vi "Laurel Meter Serial.vi"(8 "error in (no error)":errorcluster, 10 "VISA resource name":refnum<visa-resource-name>, 11 "Send Command":T1(ring)) -> (0 "error out":errorcluster, 3 "Output":dbl format="%.2f")   [LabVIEW 2012]
panel:
  out "return count":u32
  out "read buffer":string
  out "Numeric":i32
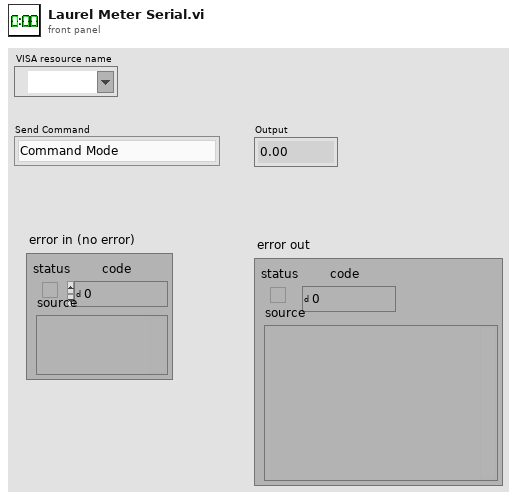
[diagram p1: front panel]
types:
  T1 = enum16{"Command Mode", "Cold Reset", "Function Reset", "Reading: All Active Items", "Reading: Item 1", "Reading: Item 2", "Reading: Item 3"}
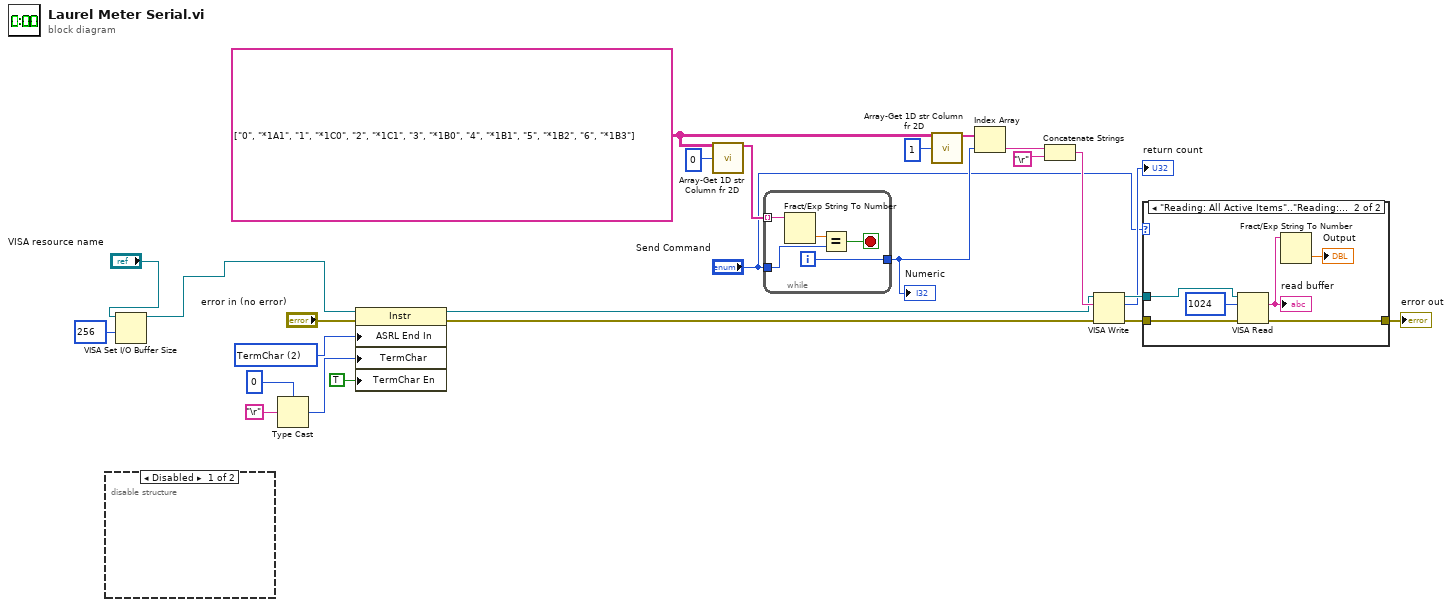
[diagram p0: block diagram]
diagram:
  w14 = u16 2 items=["None", "Last Bit", "TermChar"] ("Serial Settings:End Mode for Reads")
  w23 = string[][] [["0", "*1A1"], ["1", "*1C0"], ["2", "*1C1"], ["3", "*1B0"], ["4", "*1B1"], ["5", "*1B2"], ["6", "*1B3"]]
  n1 = disable-structure shown="Disabled" {
    frame Disabled {
    }
    frame Enabled {
    }
  }
  n2 = VISA Set I/O Buffer Size(VISA resource name="VISA resource name", size (4096)=u32 256) -> (VISA resource name out=w2:refnum<visa-resource-name>)  [unwired: 2 in, 1 out]
  n3 = Type Cast(type=u8 0, x="\r") -> (*(type *) &x=w10:u8)
  n4 = property class="Instr"(reference=w2, error in="error in (no error)", "ASRL End In"=w14, "TermChar"=w10, "TermChar En"=TRUE ("Message Based Settings:Termination Character Enable")) -> (reference out=w9:refnum<visa-resource-name>, error out=w6:errorcluster)
  n5 = call "Array-Get 1D str Column fr 2D.vi"("2D Array Data"=w23, "column index"=0) -> ("Column Data"=w24:string[])  [unwired: 13 in]
  n6 = while {
    tunnel: w24 -> [w30] mode=indexing
    tunnel: "Send Command" -> [w28]
    tunnel: [w26] -> w21
    i -> [w26]
    stop <- w27 stop-if-true
    n7 = Fract/Exp String To Number(string=w30) -> (number=w29:dbl)  [unwired: 3 in, 1 out]
    n8 = Equal?(x=w29, y=w28) -> (x = y?=w27:bool)
  }
  "Numeric" <- w21
  n9 = call "Array-Get 1D str Column fr 2D.vi"("2D Array Data"=w23, "column index"=1) -> ("Column Data"=w22:string[])  [unwired: 13 in]
  n10 = Index Array(array=w22, index=w21) -> (element=w18:string)
  n11 = Concatenate Strings(w18, "\r") -> (w16:string)
  n12 = VISA Write(VISA resource name=w9, write buffer=w16, error in (no error)=w6) -> (VISA resource name out=w19:refnum<visa-resource-name>, return count=→"return count":u32, error out=w5:errorcluster)
  n13 = case shown="\"Reading: All Active Items\"..\"Reading: Item 3\"" "Send Command" {
    tunnel: w19 -> [_ w37]
    tunnel: w5 -> [w31 w34]
    tunnel: [w31 w33] -> w4
    frame "Command Mode".."Function Reset" {
    }
    frame "Reading: All Active Items".."Reading: Item 3" {
      n14 = VISA Read(VISA resource name=w37, byte count=u32 1024, error in (no error)=w34) -> (read buffer=w35:string, error out=w33:errorcluster)  [unwired: 2 out]
      "read buffer" <- w35
      n15 = Fract/Exp String To Number(string=w35) -> (number=→"Output":dbl)  [unwired: 3 in, 1 out]
    }
  }
  "error out" <- w4
